vi "2D Bool Array To Image Data Helper.vi"(8 "Error In":errorcluster, 10 "Image Data":bool[][](array[boolean])) -> (0 "Error Out":errorcluster, 2 "Image Data":u8[](array[numeric]))   [LabVIEW 2011, in "LVH-LINX.lvlib" / "SSD1306.lvlib"]
uses:
  SSD1306.lvlib
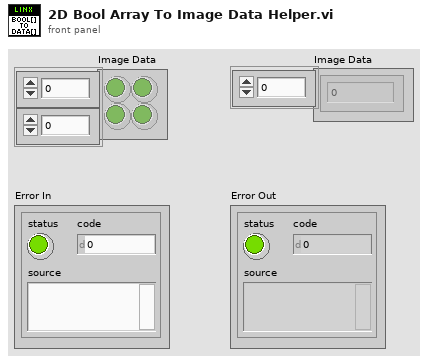
[diagram p1: front panel]
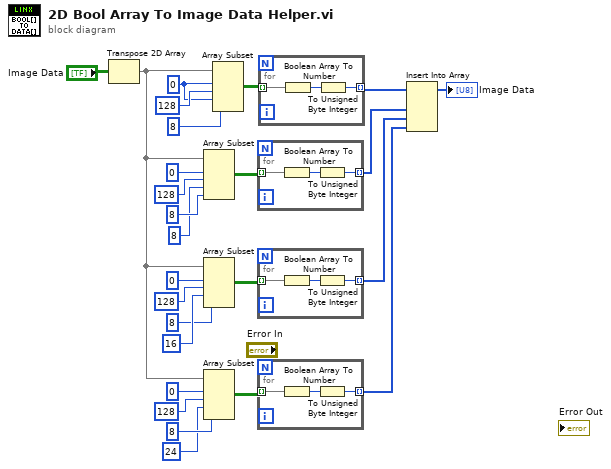
[diagram p0: block diagram]
diagram:
  w25 = 0 ("index")
  n1 = Transpose 2D Array(2D array="Image Data") -> (transposed array=w7:bool[][])
  n2 = Array Subset(array=w7, index (row)=0 ("index"), length (row)=128 ("length"), index (col)=8 ("length"), length (col)=8 ("length")) -> (w18:bool[][])
  n3 = Array Subset(array=w7, index (row)=0 ("index"), length (row)=128 ("length"), index (col)=16 ("length"), length (col)=8 ("length")) -> (w17:bool[][])
  n4 = Array Subset(array=w7, index (row)=0 ("index"), length (row)=128 ("length"), index (col)=24 ("length"), length (col)=8 ("length")) -> (w8:bool[][])
  n5 = Array Subset(array=w7, index (row)=w25, length (row)=128 ("length"), index (col)=w25, length (col)=8 ("length")) -> (w23:bool[][])
  n6 = for {
    tunnel: w18 -> [w28] mode=indexing
    tunnel: [w27] -> w5 mode=indexing
    n7 = Boolean Array To Number(Boolean array=w28) -> (number=w29:u32)
    n8 = To Unsigned Byte Integer(number=w29) -> (unsigned 8bit integer=w27:u8)
  }
  n9 = for {
    tunnel: w17 -> [w31] mode=indexing
    tunnel: [w30] -> w4 mode=indexing
    n10 = Boolean Array To Number(Boolean array=w31) -> (number=w32:u32)
    n11 = To Unsigned Byte Integer(number=w32) -> (unsigned 8bit integer=w30:u8)
  }
  n12 = for {
    tunnel: w8 -> [w34] mode=indexing
    tunnel: [w33] -> w3 mode=indexing
    n13 = Boolean Array To Number(Boolean array=w34) -> (number=w35:u32)
    n14 = To Unsigned Byte Integer(number=w35) -> (unsigned 8bit integer=w33:u8)
  }
  n15 = for {
    tunnel: w23 -> [w37] mode=indexing
    tunnel: [w36] -> w6 mode=indexing
    n16 = Boolean Array To Number(Boolean array=w37) -> (number=w38:u32)
    n17 = To Unsigned Byte Integer(number=w38) -> (unsigned 8bit integer=w36:u8)
  }
  n18 = Insert Into Array(array=w6, new element #1=w5, new element #2=w4, new element #3=w3) -> (→"Image Data":u8[])  [unwired: 1 in]
